vi "testCreateElement.vi"(8 "error in (no error)":errorcluster) -> (0 "error out":errorcluster)   [LabVIEW 2018]
uses:
  SALTypeGenerator/ElementFactory/ElementFactory/ElementFactory.lvclass
  SALTypeGenerator/Typedefs/CollectionInfo.ctl
  SALTypeGenerator/Elements/Array/Array.lvclass
  SALTypeGenerator/Elements/Enum/Enum.lvclass
  SALTypeGenerator/Elements/Array/Array.lvclass/Array.ctl
  SALTypeGenerator/Elements/Enum/Enum.lvclass/Enum.ctl
  SALTypeGenerator/Element/Element.lvclass/Element.ctl
  <vilib>/addons/_JKI Toolkits/Caraya/classes/Assert/Assert Equal Value_Variant.vi
  SALTypeGenerator/Elements/Primitive/Primitive.lvclass
  <vilib>/addons/_JKI Toolkits/Caraya/classes/Test/Test.lvclass
  <vilib>/addons/_JKI Toolkits/Caraya/classes/Assert/Assert.lvclass
  SALTypeGenerator/Element/Element.lvclass
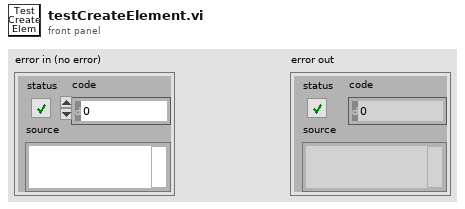
[diagram p1: front panel]
types:
  T1 = typedef "CollectionInfo.ctl" = cluster{"isArray?":bool, "arraySize":u16}
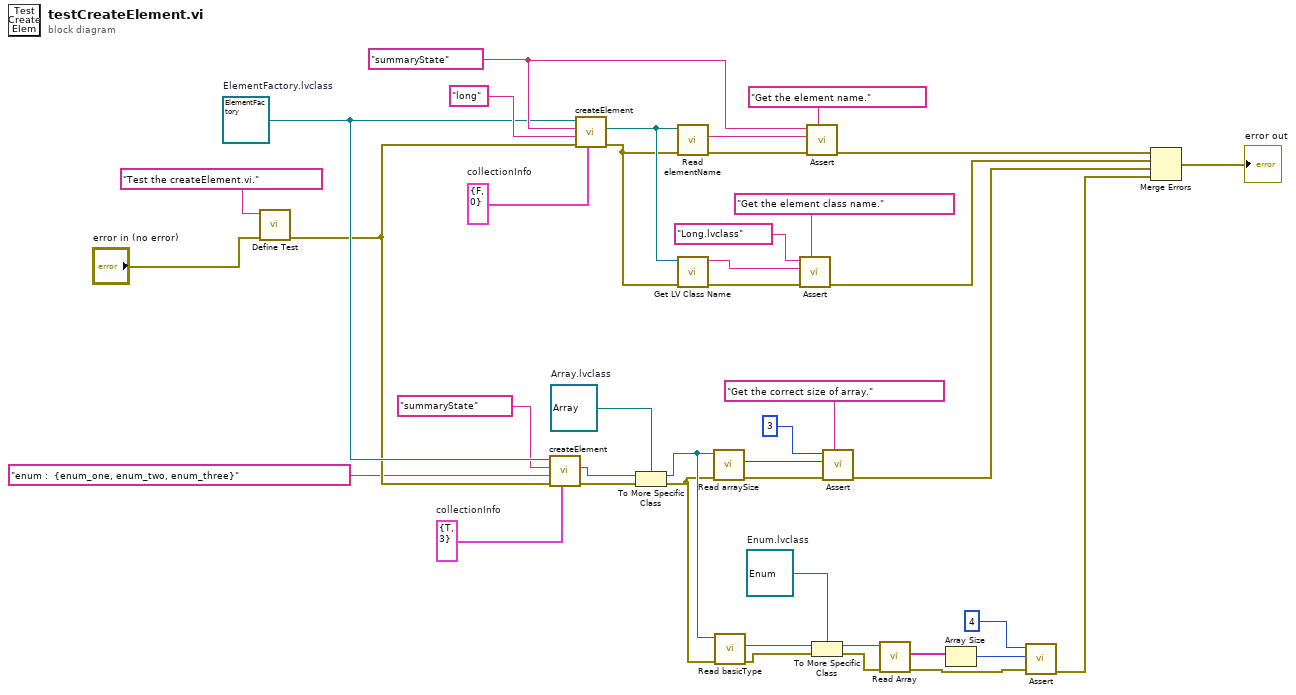
[diagram p0: block diagram]
diagram:
  w9 = refnum<class "Enum.lvclass"> refnum  # Enum.lvclass
  w20 = refnum<class "Array.lvclass"> refnum  # Array.lvclass
  w21 = T1 {"isArray?"=TRUE, "arraySize"=3}  # collectionInfo
  w41 = T1 {"isArray?"=FALSE, "arraySize"=0}  # collectionInfo
  w36 = "summaryState" ("elementName")
  w25 = refnum<class "ElementFactory.lvclass"> refnum  # ElementFactory.lvclass
  n1 = call <vilib>:"Define Test.vi"("error in (no error)"="error in (no error)", "Label (VI Title)"="Test the createElement.vi.") -> ("error out"=w24:errorcluster)  [unwired: 9 in]
  n2 = call-dynamic "createElement.vi"("collectionInfo"=w21, "error in (no error)"=w24, "elementBasicType"="enum :  {enum_one, enum_two, enum_three}", "elementName"="summaryState", "ElementFactory in"=w25) -> ("error out"=w15:errorcluster, "element"=w14:refnum<class "Element.lvclass">)  [unwired: 4 in, 1 out]
  n3 = call-dynamic "createElement.vi"("collectionInfo"=w41, "error in (no error)"=w24, "elementBasicType"="long", "elementName"=w36, "ElementFactory in"=w25) -> ("error out"=w33:errorcluster, "element"=w34:refnum<class "Element.lvclass">)  [unwired: 4 in, 1 out]
  n4 = To More Specific Class(target class=w20, reference=w14, error in=w15) -> (specific class reference=w12:refnum<class "Array.lvclass">, error out=w11:errorcluster)
  n5 = call "Read elementName.vi"("error in (no error)"=w33, "Element in"=w34) -> ("error out"=w38:errorcluster, "elementName"=w37:string)  [unwired: 7 in, 1 out]
  n6 = call <vilib>:"Get LV Class Name.vi"("error in (no error)"=w33, "object"=w34) -> ("error out"=w32:errorcluster, "class name"=w31:string)  [unwired: 8 in]
  n7 = call "Read arraySize.vi"("error in (no error)"=w11, "Array in"=w12) -> ("error out"=w19:errorcluster, "arraySize"=w18:u16)  [unwired: 7 in, 1 out]
  n8 = call "Read basicType.vi"("error in (no error)"=w11, "Array in"=w12) -> ("error out"=w8:errorcluster, "Primitive.lvclass"=w10:refnum<class "Primitive.lvclass">)  [unwired: 7 in, 1 out]
  n9 = call-poly <vilib>:"Assert.vi"("Label"="Get the element class name.", "error in (no error)"=w32, "Y"=w31, "X"="Long.lvclass" ("Label")) -> ("error out"=w26:errorcluster)  [unwired: 7 in]
  n10 = call-poly <vilib>:"Assert.vi"("Label"="Get the element name.", "error in (no error)"=w38, "Y"=w37, "X"=w36) -> ("error out"=w28:errorcluster)  [unwired: 7 in]
  n11 = To More Specific Class(target class=w9, reference=w10, error in=w8) -> (specific class reference=w7:refnum<class "Enum.lvclass">, error out=w5:errorcluster)
  n12 = call-poly <vilib>:"Assert.vi"("Label"="Get the correct size of array.", "error in (no error)"=w19, "Y"=w18, "X"=3) -> ("error out"=w13:errorcluster)  [unwired: 7 in]
  n13 = call "Read Array.vi"("error in (no error)"=w5, "Enum in"=w7) -> ("error out"=w3:errorcluster, "Array"=w6:string[])  [unwired: 7 in, 1 out]
  n14 = Array Size(array=w6) -> (size(s)=w4:i32)
  n15 = call-poly <vilib>:"Assert.vi"("error in (no error)"=w3, "Y"=w4, "X"=4) -> ("error out"=w1:errorcluster)  [unwired: 8 in]
  n16 = Merge Errors(w28, w26, w13, w1) -> (→"error out":errorcluster)
